vi "FrontPanelSingleChannel.vi"() -> ()   [LabVIEW 2017, in "LD Reading.lvclass"]
uses:
  LD Reading.lvclass
  Experimental Parameters.ctl
  Reference Channel Intensities.ctl
  Sample Channel Intensities.ctl
  Realtime Output.ctl
  Average Data.ctl
  AmplifierSettings.ctl
  LD Reading.lvclass/LD Reading.ctl
  MCTypedef.ctl
  <vilib>/Instr/_visa.llb/VISA Configure Serial Port (Instr).vi
  <vilib>/Utility/file.llb/Write Delimited Spreadsheet (string).vi
  <vilib>/Utility/inputDevices.llb/keyboardAcquire.vi
panel:
  in  "Experimental Controls":T1(tab)
  in  "Measure Dark Current":bool
  in  "Collect Data":bool
  out "Running":bool
  in  "Save Measurements?":bool
  in  "Stop and Discard \nMeasurement":bool
  in  "Output Filename (stem)":path
  out "Finished":bool
  in  "Data Collection Mode":enum32{"Reference", "Sample"}(radio)
  in  "Export Data":bool
  in  "Experimental Parameters":T2={"Correction Factor"=2.9405, "Data Interval (s)"=1.0, "Number of Data Points"=60.0, "Incident Angle (Degrees)"=63.0, "Refractive Index (Rare)"=1.335, "Refractive Index (Dense)"=1.55222, "PMT Bias Voltage (V)"=0.0, "Laser Wavelength (nm)"=0.0, "Preamplifier Output Gain (uA/V)"=10.0, "PEM Monitoring Frequency"=2} {"PEM Monitoring Frequency" min=1 max=2 step=1}
  in  "stop":bool
  out "read buffer":string
  in  "sp33d":dbl(knob)=0.5 step=0.5 scale=0.5..1.0
  in  "clear":bool
  out "error out":errorcluster
  out "Status":string
  out "Data Collection Progress":u8(slide) scale=0.0..100.0
  out "Reference Amplifier Settings":T3
  out "Signal Amplifier Settings":T3
  out "Corrected Signal":cluster{dbl[], dbl[]}(graph)
  out "RMS Voltage":cluster{dbl[], dbl[]}(graph)
  out "Signal PMT Voltage":cluster{dbl[], dbl[]}(graph)
  out "Reference PMT Voltage":cluster{dbl[], dbl[]}(graph)
  out "Realtime Output":T4
  out "Reference Averages":T5
  out "Sample Averages":T5
  out "Reference Analysis":T6
  out "Sample Analysis":T7
  # "Dichroism Controller"
  # "Translation Stage Controls"
  # "Data Collection Parameters"
  # "System Settings"
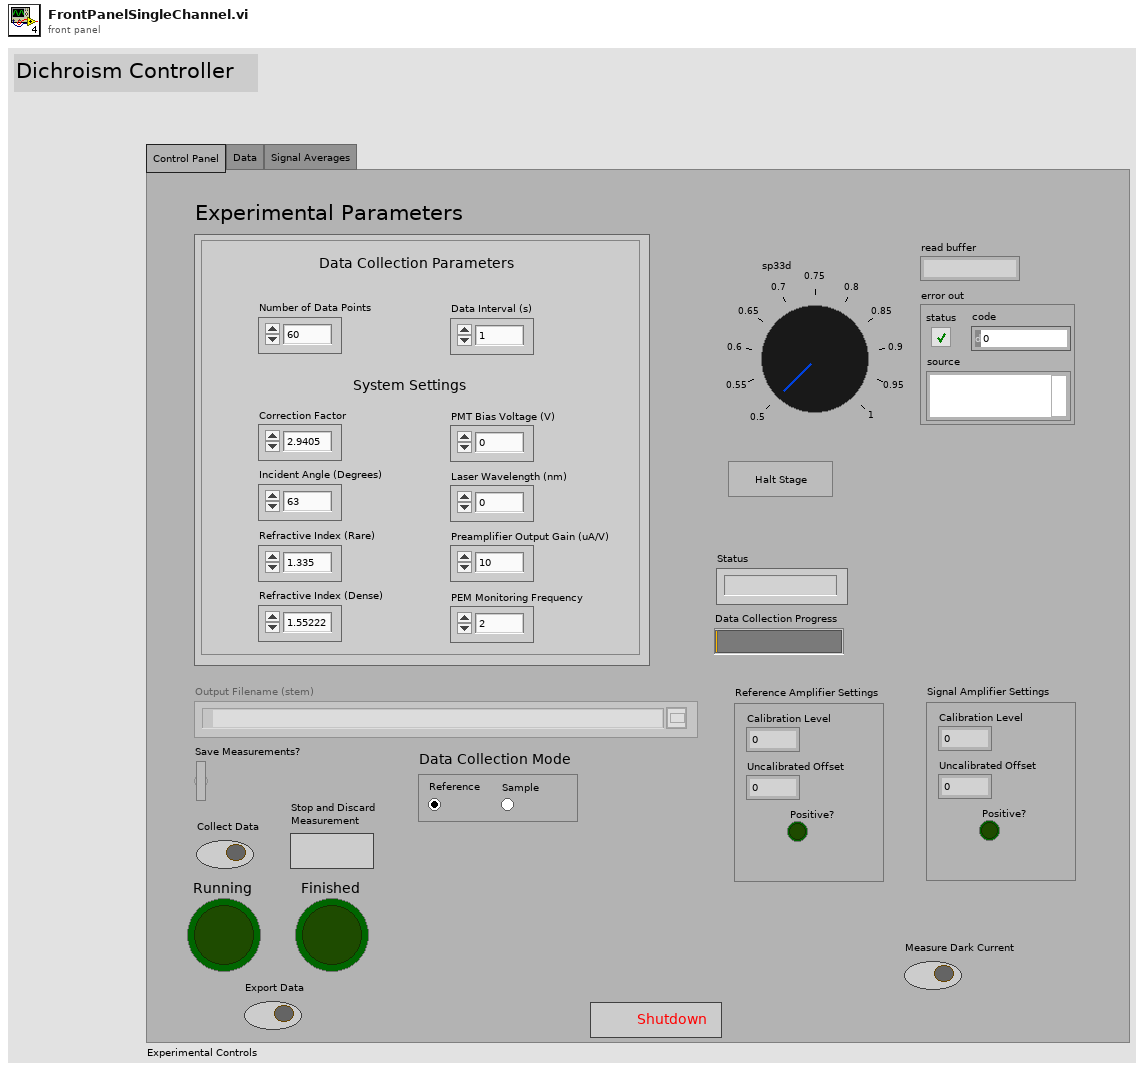
[diagram p1: front panel]
types:
  T1 = enum32{"Control Panel", "Data", "Signal Averages"}
  T2 = typedef "Experimental Parameters.ctl" = cluster{"Correction Factor":dbl, "Data Interval (s)":dbl, "Number of Data Points":dbl, "Incident Angle (Degrees)":dbl, "Refractive Index (Rare)":dbl, "Refractive Index (Dense)":dbl, "PMT Bias Voltage (V)":dbl, "Laser Wavelength (nm)":dbl, "Preamplifier Output Gain (uA/V)":dbl, "PEM Monitoring Frequency":u8}
  T3 = typedef "AmplifierSettings.ctl" = cluster{"Calibration Level":dbl, "Uncalibrated Offset":dbl, "Positive?":bool}
  T4 = typedef "Realtime Output.ctl" = cluster{"Elapsed Time (s)":dbl, "PMT Voltage (V)":dbl, "Diode Voltage (V)":dbl, "RMS Voltage (V)":dbl, "Theta (Degrees)":dbl, "PEM Frequency (Hz)":dbl}
  T5 = typedef "Average Data.ctl" = cluster{"Data":cluster{"Signal PMT Voltage (V)":dbl, "Reference PMT Voltage (V)":dbl, "RMS Voltage (V)":dbl, "Theta (Degrees)":dbl}}
  T6 = typedef "Reference Channel Intensities.ctl" = cluster{"Data":cluster{"I_par":dbl, "I_perp":dbl}}
  T7 = typedef "Sample Channel Intensities.ctl" = cluster{"Data":cluster{"I_par":dbl, "I_perp":dbl, "Dichroic Ratio":dbl, "Angle (Degrees)":dbl}}
  T8 = enum8{"Enabled", "Disabled", "Disabled and Grayed Out"}
  T9 = typedef "MCTypedef.ctl" = enum16{"idle", "forward", "reverse", "clear"}
  T10 = cluster{dbl[], dbl[], dbl[], dbl[], dbl[], dbl[], dbl[]}
  T11 = cluster{"RMS Voltage Array":dbl[], "Photodiode Voltage Array":dbl[], "PMT Voltage Array":dbl[], "Diode/PMT Ratio Array":dbl[], "Time Array":dbl[], "PEM Frequency Array":dbl[], "Theta Array":dbl[]}
  T12 = cluster{"Signal PMT Voltage (V)":dbl, "Reference PMT Voltage (V)":dbl, "RMS Voltage (V)":dbl, "Theta (Degrees)":dbl}
  T13 = cluster{"I_par":dbl, "I_perp":dbl, "Dichroic Ratio":dbl, "Angle (Degrees)":dbl}
  T14 = typedef "NI_Matrix.lvlib/RealMatrix.ctl" = dbl[][]
  T15 = enum16{"0", "1", "2", "3", "4", "5", "6", "7", "8", "9", "A", "B", "C", "D", "E", "F", "G", "H", "I", "J", "K", "L", "M", "N", "O", "P", "Q", "R", "S", "T", "U", "V", "W", "X", "Y", "Z", "F1", "F2", "F3", "F4", "F5", "F6", "F7", "F8", "F9", "F10", "F11", "F12", "F13", "F14", "F15", "ADD", "BACK", "BACKSLASH", "CAPITAL", "COMMA", "DECIMAL", "DELETE", "DIVIDE", "DOWN", "END", "EQUALS", "ESCAPE", "GRAVE (`)", "HOME", "INSERT", "LBRACKET", "LCONTROL", "LEFT", "L ALT", "LSHIFT", "LWIN", "MINUS", "MULTIPLY", "NEXT", "NUMLOCK", "NUMPAD_0", "NUMPAD_1", "NUMPAD_2", "NUMPAD_3", "NUMPAD_4", "NUMPAD_5", "NUMPAD_6", "NUMPAD_7", "NUMPAD_8", "NUMPAD_9", "PAUSE", "PERIOD", "PRIOR (PG UP)", "RBRACKET", "RCONTROL", "RETURN", "RIGHT", "R ALT", "RSHIFT", "RWIN", "SCROLL", "SEMICOLON", "SLASH", "SPACE", "SUBTRACT", "TAB", "UP", "ENTER (num pad)", "' (quote)"}[]
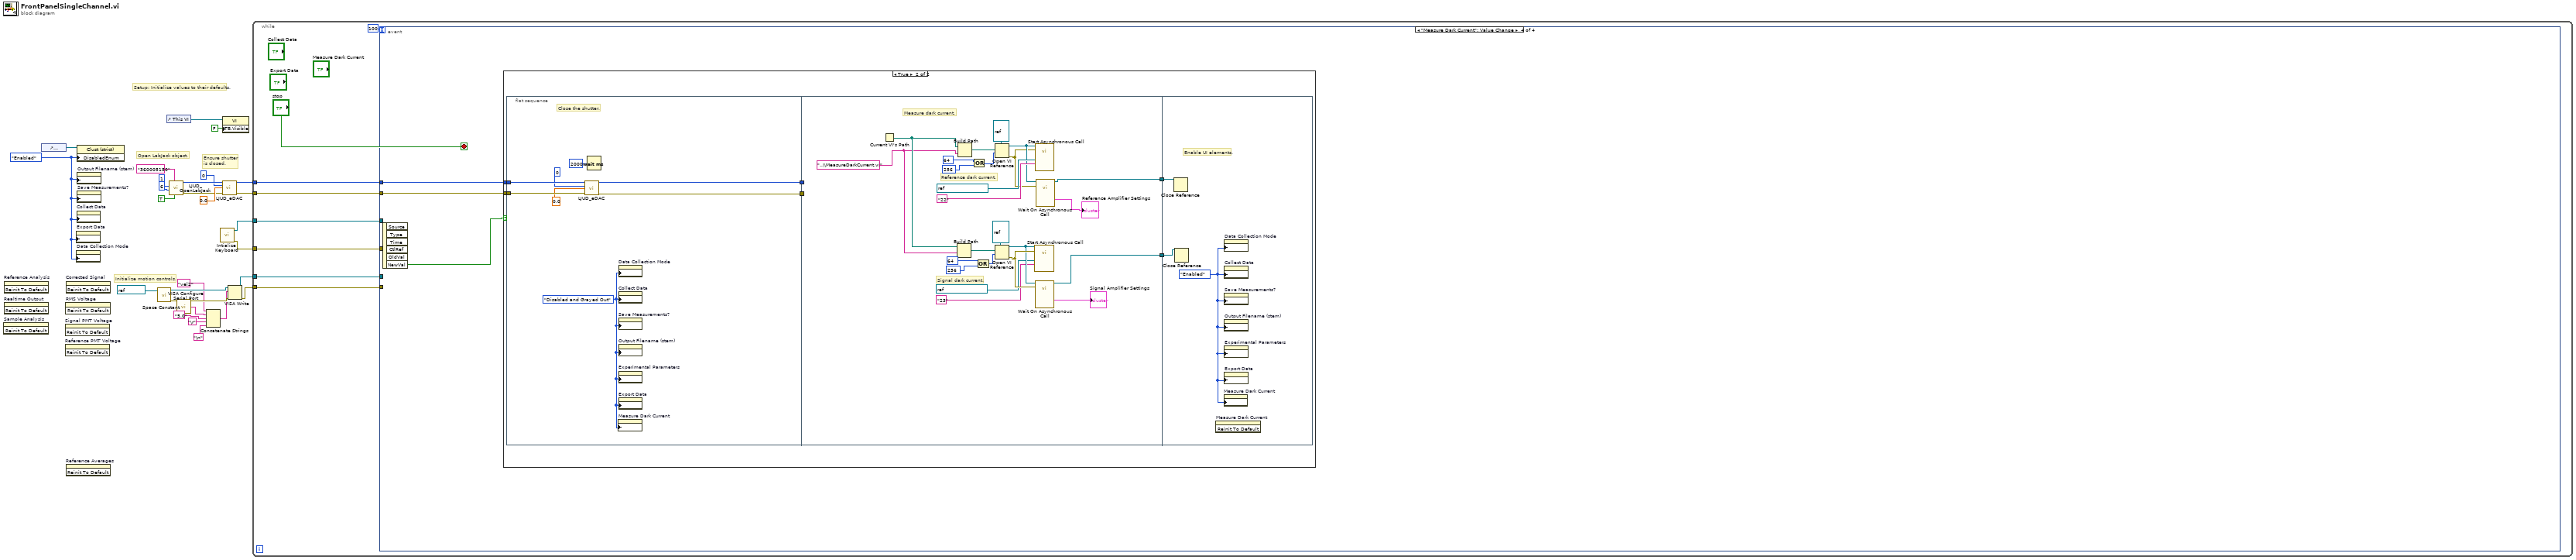
[diagram p0: block diagram]
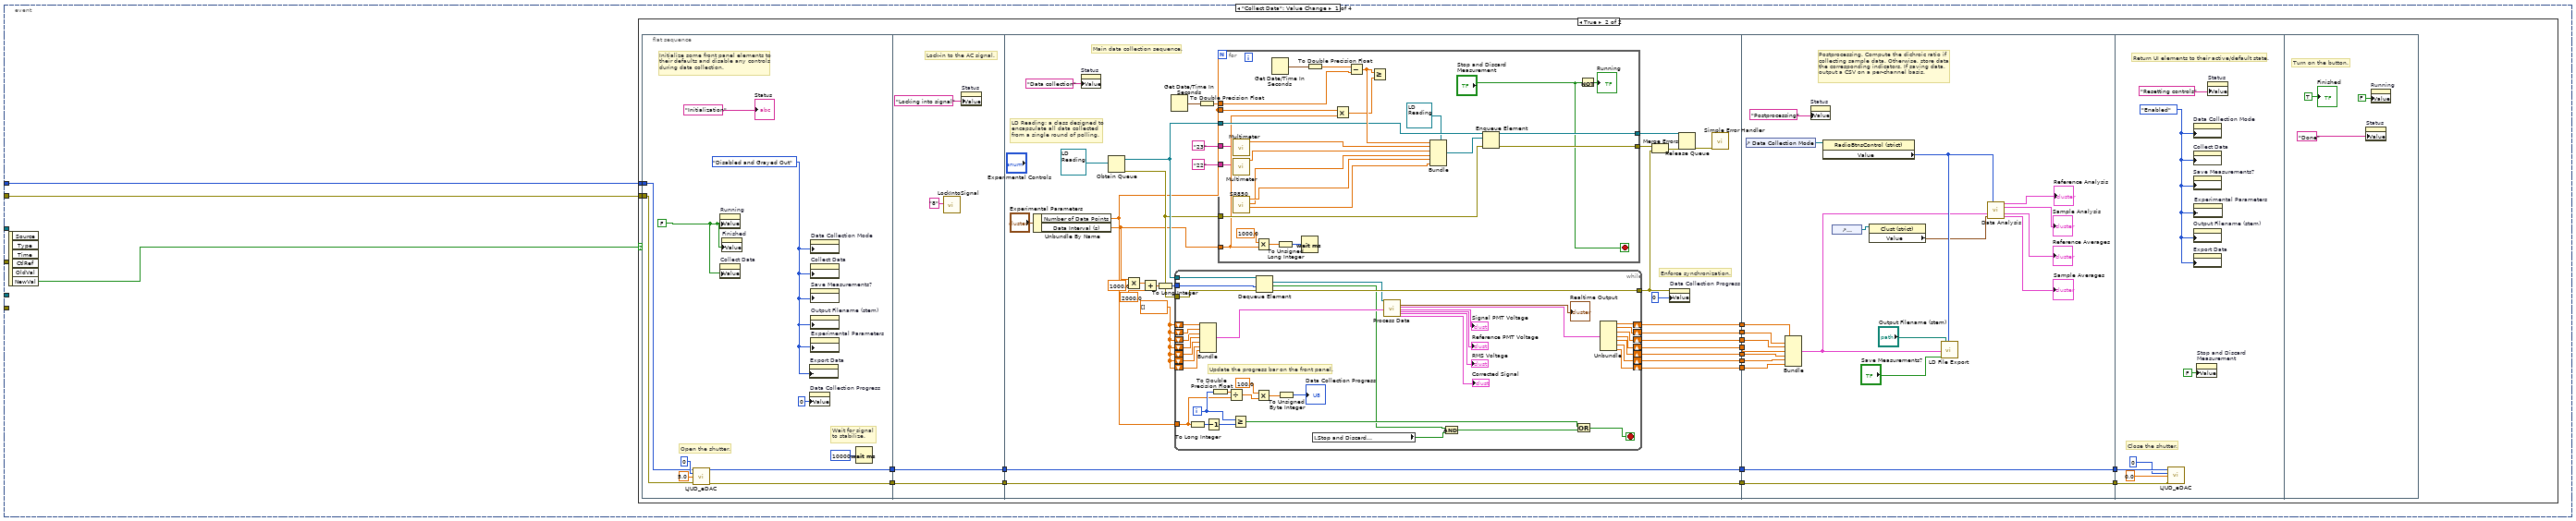
[diagram p2: hidden frame]
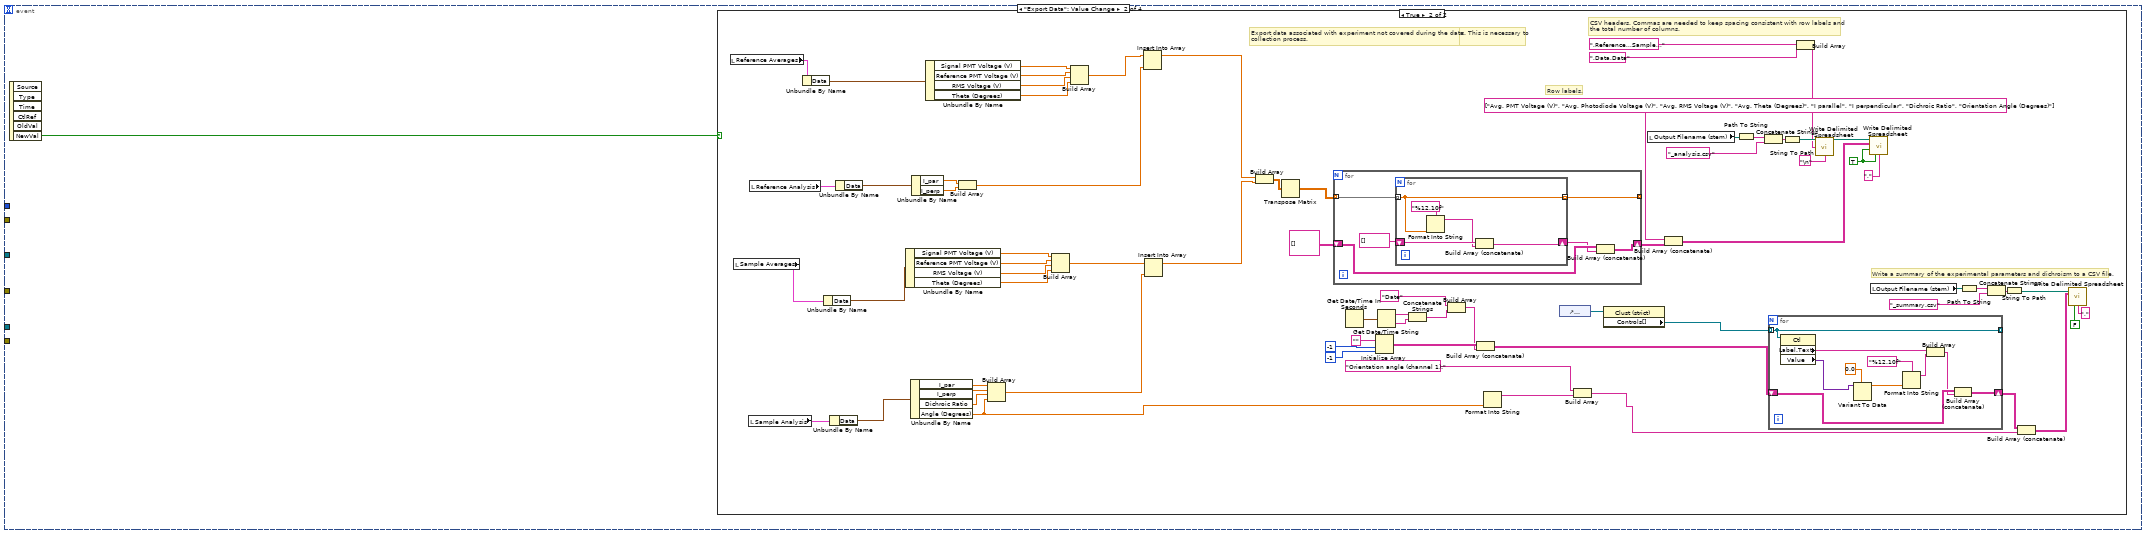
[diagram p4: hidden frame]
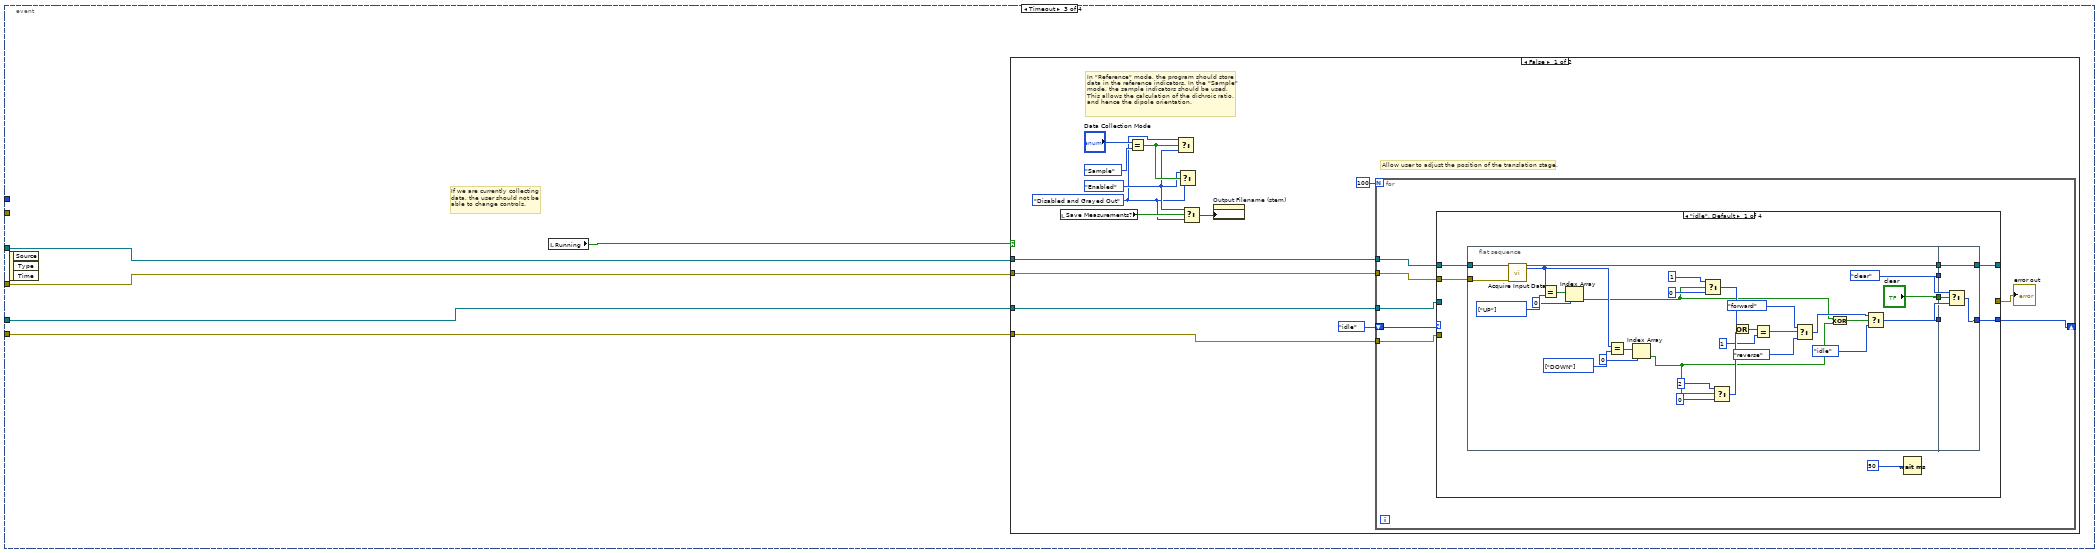
[diagram p6: hidden frame]
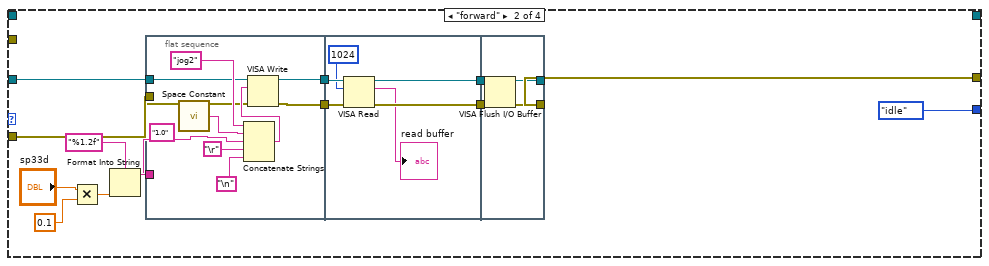
[diagram p7: hidden frame]
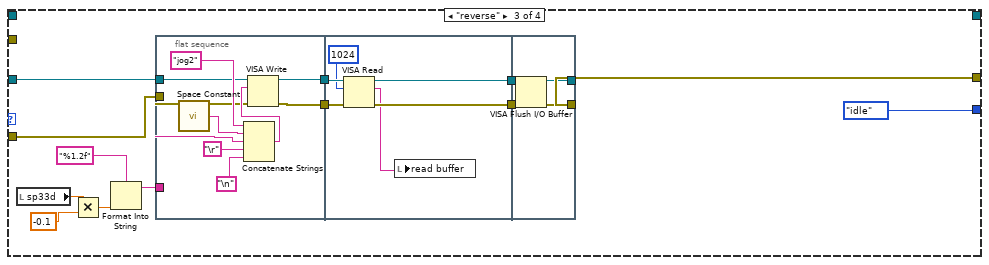
[diagram p8: hidden frame]
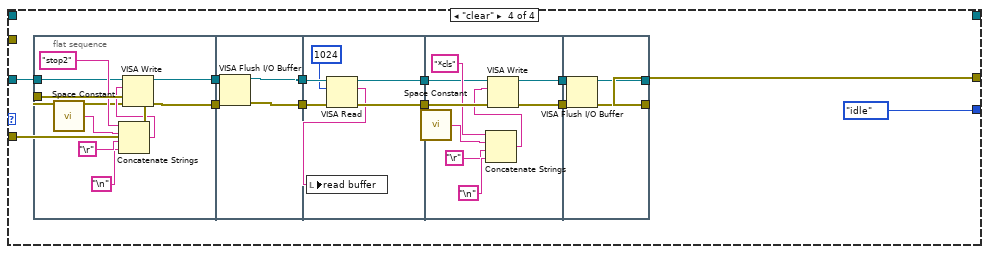
[diagram p9: hidden frame]
diagram:
  w24 = T8."Enabled" ("Disabled")
  # "Ensure shutter\nis closed."
  # "Open LabJack object."
  # "Initialize motion controls."
  # "Setup: Initialize values to their defaults."
  n1 = invoke on="Sample Analysis" class="Clust (strict)" method="Reinit To Default"() -> ()  [unwired: 3 in, 3 out]
  n2 = invoke on="Reference Analysis" class="Clust (strict)" method="Reinit To Default"() -> ()  [unwired: 3 in, 3 out]
  n3 = invoke on="Realtime Output" class="Clust (strict)" method="Reinit To Default"() -> ()  [unwired: 3 in, 3 out]
  n4 = control-ref of="Experimental Parameters"() -> (w25:refnum<vi>)
  n5 = invoke on="Signal PMT Voltage" class="XYGraph (strict)" method="Reinit To Default"() -> ()  [unwired: 3 in, 3 out]
  n6 = invoke on="Reference PMT Voltage" class="XYGraph (strict)" method="Reinit To Default"() -> ()  [unwired: 3 in, 3 out]
  n7 = invoke on="RMS Voltage" class="XYGraph (strict)" method="Reinit To Default"() -> ()  [unwired: 3 in, 3 out]
  n8 = invoke on="Corrected Signal" class="XYGraph (strict)" method="Reinit To Default"() -> ()  [unwired: 3 in, 3 out]
  n9 = invoke on="Reference Averages" class="Clust (strict)" method="Reinit To Default"() -> ()  [unwired: 3 in, 3 out]
  n10 = property on="Export Data" class="Bool"("DisabledEnum"=w24) -> ()  [unwired: 2 in, 2 out]
  n11 = property on="Data Collection Mode" class="RadioBtnsControl (strict)"("DisabledEnum"=w24) -> ()  [unwired: 2 in, 2 out]
  n12 = property class="Clust (strict)"(reference=w25, "DisabledEnum"=w24) -> ()  [unwired: 1 in, 2 out]
  n13 = property on="Collect Data" class="Bool (strict)"("DisabledEnum"=w24) -> ()  [unwired: 2 in, 2 out]
  n14 = property on="Output Filename (stem)" class="Path"("DisabledEnum"=w24) -> ()  [unwired: 2 in, 2 out]
  n15 = property on="Save Measurements?" class="Bool (strict)"("DisabledEnum"=w24) -> ()  [unwired: 2 in, 2 out]
  n16 = call-poly "VISA Configure Serial Port"("VISA resource name"=refnum<visa-resource-name> "COM1") -> ("VISA resource name out"=w22:refnum<visa-resource-name>, "error out"=w23:errorcluster)  [unwired: 13 in]
  n17 = control-ref of="This VI"() -> (w26:refnum<vi>)
  n18 = call "LJUD_OpenLabJack.vi"("FirstFound"=TRUE, "Address"="360005150", "ConnectionType"=1, "DeviceType"=6) -> ("error out"=w1:errorcluster, "Handle"=w6:i32)  [unwired: 6 in]
  n19 = call <vilib>:"Space Constant.vi"() -> ("String"=w21:string)
  n20 = Concatenate Strings("vel2" ("string"), w21, "5.0" ("string"), "\r", "\n") -> (w20:string)
  n21 = call <vilib>:"Intialize Keyboard.vi"() -> ("error out"=w12:errorcluster, "device ID"=w11:refnum<k1>)  [unwired: 10 in]
  n22 = property class="VI"(reference=w26, "TB.Visible"=FALSE ("Tool Bar:Visible")) -> ()  [unwired: 1 in, 2 out]
  n23 = call "LJUD_eDAC.vi"("Handle In"=w6, "Channel"=0, "Voltage"=0.0, "error in"=w1) -> ("Handle Out"=w5:i32, "error out"=w4:errorcluster)  [unwired: 10 in]
  n24 = VISA Write(VISA resource name=w22, write buffer=w20, error in (no error)=w23) -> (VISA resource name out=w13:refnum<visa-resource-name>, error out=w14:errorcluster)  [unwired: 1 out]
  n25 = while {
    tunnel: w14 -> [w33]
    tunnel: w13 -> [w32]
    tunnel: w12 -> [w31]
    tunnel: w11 -> [w30]
    tunnel: w5 -> [w29]
    tunnel: w4 -> [w28]
    stop <- "stop" stop-if-true
    n26 = event shown="[3] \"Measure Dark Current\": Value Change" {
      selector: _ -> [_ _ _ _]
      dyn-events: _ -> [_ _ _ _]
      timeout: 100 -> [_ _ _ _]
      tunnel: w33 -> [_ _ w295 _]
      tunnel: w32 -> [_ _ w294 _]
      tunnel: w31 -> [_ _ w293 _]
      tunnel: w30 -> [_ _ w292 _]
      tunnel: w29 -> [w37 _ _ w471]
      tunnel: w28 -> [w36 _ _ w470]
      event "Collect Data": Value Change {
        n27 = event-data() -> ("NewVal"=w38:bool)  [unwired: 1 in, 5 out]
        n28 = case shown="True" w38 {
          tunnel: w37 -> [_ w48]
          tunnel: w36 -> [_ w47]
          frame False {
          }
          frame True {
            n29 = flat-sequence {
              tunnel: w48 -> [w60]
              tunnel: w47 -> [w59]
              tunnel: [w58] -> w42
              tunnel: [w57] -> w40
              tunnel: w42 -> [w70]
              tunnel: [w70] -> w41
              tunnel: w40 -> [w69]
              tunnel: [w69] -> w39
              tunnel: [w92] -> w55
              tunnel: [w91] -> w54
              tunnel: [w90] -> w53
              tunnel: [w93] -> w52
              tunnel: [w89] -> w51
              tunnel: [w88] -> w50
              tunnel: [w83] -> w49
              tunnel: [w72] -> w45
              tunnel: w41 -> [w72]
              tunnel: [w71] -> w43
              tunnel: w39 -> [w71]
              tunnel: w55 -> [w184]
              tunnel: w54 -> [w183]
              tunnel: w53 -> [w182]
              tunnel: w52 -> [w185]
              tunnel: w51 -> [w181]
              tunnel: w50 -> [w180]
              tunnel: w49 -> [w179]
              tunnel: [w169] -> w46
              tunnel: w45 -> [w169]
              tunnel: [w168] -> w44
              tunnel: w43 -> [w168]
              tunnel: w46 -> [w192]
              tunnel: w44 -> [w191]
              frame #0 {
                w63 = T8."Disabled and Grayed Out" ("Disabled")
                w64 = FALSE
                # "Wait for signal \nto stabilize."
                # "Open the shutter."
                # "Initialize some front panel elements to \ntheir defaults and disable any controls \nduring data collection."
                n30 = call "LJUD_eDAC.vi"("Handle In"=w60, "Channel"=0, "Voltage"=5.0, "error in"=w59) -> ("Handle Out"=w58:i32, "error out"=w57:errorcluster)  [unwired: 10 in]
                n31 = property on="Running" class="Bool (strict)"("Value"=w64) -> ()  [unwired: 2 in, 2 out]
                n32 = property on="Collect Data" class="Bool (strict)"("Value"=w64) -> ()  [unwired: 2 in, 2 out]
                n33 = property on="Finished" class="Bool (strict)"("Value"=w64) -> ()  [unwired: 2 in, 2 out]
                n34 = property on="Export Data" class="Bool"("DisabledEnum"=w63) -> ()  [unwired: 2 in, 2 out]
                n35 = property on="Data Collection Progress" class="Slide (strict)"("Value"=u8 0 ("Progress")) -> ()  [unwired: 2 in, 2 out]
                n36 = property on="Data Collection Mode" class="RadioBtnsControl (strict)"("DisabledEnum"=w63) -> ()  [unwired: 2 in, 2 out]
                n37 = property on="Collect Data" class="Bool (strict)"("DisabledEnum"=w63) -> ()  [unwired: 2 in, 2 out]
                n38 = property on="Save Measurements?" class="Bool (strict)"("DisabledEnum"=w63) -> ()  [unwired: 2 in, 2 out]
                n39 = property on="Output Filename (stem)" class="Path"("DisabledEnum"=w63) -> ()  [unwired: 2 in, 2 out]
                n40 = property on="Experimental Parameters" class="Clust (strict)"("DisabledEnum"=w63) -> ()  [unwired: 2 in, 2 out]
                n41 = Wait (ms)(milliseconds to wait=u32 10000) -> ()  [unwired: 1 out]
                "Status" <- "Initialization"
              }
              frame #1 {
                # "Lock-in to the AC signal."
                n42 = call "LockIntoSignal.vi"("GPIB Address"="8") -> ()  [unwired: 10 in, 1 out]
                n43 = property on="Status" class="Str"("Value"="Locking into signal") -> ()  [unwired: 2 in, 2 out]
              }
              frame #2 {
                w84 = dbl[] []
                # "Enforce synchronization."
                # "Main data collection sequence."
                # "LD Reading: a class designed to \nencapsulate all data collected \nfrom a single round of polling."
                n44 = Unbundle By Name("Experimental Parameters") -> ("Number of Data Points"=w81:dbl, "Data Interval (s)"=w80:dbl)
                n45 = property on="Status" class="Str"("Value"="Data collection") -> ()  [unwired: 2 in, 2 out]
                n46 = Obtain Queue(element data type=refnum<class "LD Reading.lvclass"> refnum ("LD Reading.lvclass")) -> (queue out=w99:refnum<queue>, error out=w98:errorcluster)  [unwired: 4 in, 1 out]
                n47 = Multiply(x=w80, y=1000.0) -> (x*y=w78:dbl)
                n48 = Add(x=w78, y=2000.0) -> (x+y=w76:dbl)
                n49 = To Long Integer(number=w76) -> (32bit integer=w75:i32)
                n50 = Get Date/Time In Seconds() -> (seconds since 1Jan1904=w102:timestamp)
                n51 = while {
                  tunnel: w99 -> [w167]
                  shift-right: [w146] -> w93
                  shift-left: w84 -> [w153]
                  shift-right: [w145] -> w92
                  shift-left: w84 -> [w152]
                  shift-right: [w144] -> w91
                  shift-left: w84 -> [w151]
                  shift-right: [w143] -> w90
                  shift-left: w84 -> [w150]
                  shift-right: [w142] -> w89
                  shift-left: w84 -> [w149]
                  shift-right: [w141] -> w88
                  shift-left: w84 -> [w148]
                  shift-right: [w140] -> w83
                  shift-left: w84 -> [w147]
                  tunnel: w98 -> [w165]
                  tunnel: [w164] -> w86
                  tunnel: w81 -> [w154]
                  tunnel: w75 -> [w128]
                  i -> [w159]
                  stop <- w166 stop-if-true
                  # "Update the progress bar on the front panel."
                  n52 = To Long Integer(number=w154) -> (32bit integer=w160:i32)
                  n53 = Bundle(w153, w152, w151, w150, w149, w148, w147) -> (w138:T10)  [unwired: 1 in]
                  n54 = Decrement(x=w160) -> (x-1=w163:i32)
                  n55 = To Double Precision Float(number=w159) -> (double precision float=w158:dbl)
                  n56 = Divide(x=w158, y=w154) -> (x/y=w161:dbl)
                  n57 = Greater Or Equal?(x=w159, y=w163) -> (x >= y?=w162:bool)
                  n58 = Multiply(x=100.0, y=w161) -> (x*y=w156:dbl)
                  n59 = Dequeue Element(queue=w167, timeout in ms (-1)=w128, error in (no error)=w165) -> (element=w139:refnum<class "LD Reading.lvclass">, timed out?=w131:bool, error out=w164:errorcluster)  [unwired: 1 out]
                  n60 = To Unsigned Byte Integer(number=w156) -> (unsigned 8bit integer=→"Data Collection Progress":u8)
                  n61 = local read "Stop and Discard \nMeasurement"() -> (w130:bool)
                  n62 = call "Process Data.vi"("LD Reading in"=w139, "Input Cluster"=w138) -> ("Realtime Output"=→"Realtime Output":T4, "Output Cluster"=w136:T11, "PMT Voltage (V)"=→"Signal PMT Voltage":cluster{dbl[], dbl[]}, "Photodiode Voltage  (V)"=→"Reference PMT Voltage":cluster{dbl[], dbl[]}, "RMS Voltage (mV)"=→"RMS Voltage":cluster{dbl[], dbl[]}, "Diode/PMT"=→"Corrected Signal":cluster{dbl[], dbl[]})  [unwired: 20 in]
                  n63 = And(x=w131, y=w130) -> (x .and. y?=w129:bool)
                  n64 = Or(x=w162, y=w129) -> (x .or. y?=w166:bool)
                  n65 = Unbundle(w136) -> ("RMS Voltage Array"=w146:dbl[], "Photodiode Voltage Array"=w145:dbl[], "PMT Voltage Array"=w144:dbl[], "Diode/PMT Ratio Array"=w143:dbl[], "Time Array"=w142:dbl[], "PEM Frequency Array"=w141:dbl[], "Theta Array"=w140:dbl[])
                }
                n66 = To Double Precision Float(number=w102) -> (double precision float=w101:dbl)
                n67 = for {
                  N: w81 -> [_]
                  tunnel: w80 -> [w108]
                  tunnel: w101 -> [w117]
                  tunnel: w99 -> [w124]
                  tunnel: [w121] -> w94
                  tunnel: w98 -> [w119]
                  tunnel: [w118] -> w97
                  tunnel: w81 -> [w116]
                  tunnel: "23" ("GPIB Address") -> [w105]
                  tunnel: "22" ("GPIB Address") -> [w103]
                  stop <- "Stop and Discard \nMeasurement" stop-if-true
                  n68 = call "Multimeter.vi"("GPIB Address"=w105) -> ("Voltage"=w111:dbl)  [unwired: 9 in, 1 out]
                  n69 = call "Multimeter.vi"("GPIB Address"=w103) -> ("Voltage"=w104:dbl)  [unwired: 9 in, 1 out]
                  n70 = call "SR850.vi"() -> ("Frequency"=w112:dbl, "R"=w113:dbl, "Theta"=w114:dbl)  [unwired: 8 in, 1 out]
                  n71 = Multiply(x=1000.0, y=w108) -> (x*y=w110:dbl)
                  n72 = Get Date/Time In Seconds() -> (seconds since 1Jan1904=w127:timestamp)
                  n73 = To Unsigned Long Integer(number=w110) -> (unsigned 32bit integer=w107:u32)
                  n74 = Wait (ms)(milliseconds to wait=w107) -> ()  [unwired: 1 out]
                  n75 = To Double Precision Float(number=w127) -> (double precision float=w126:dbl)
                  n76 = Multiply(x=w116, y=w108) -> (x*y=w115:dbl)
                  n77 = Subtract(x=w126, y=w117) -> (x-y=w125:dbl)
                  n78 = Greater Or Equal?(x=w125, y=w115) -> ()  [unwired: 1 out]
                  n79 = Bundle(cluster=refnum<class "LD Reading.lvclass"> refnum ("LD Reading.lvclass"), w125, w111, w104, w113, w114, w112) -> (w122:refnum<class "LD Reading.lvclass">)
                  n80 = Enqueue Element(queue=w124, element=w122, error in (no error)=w119) -> (queue out=w121:refnum<queue>, error out=w118:errorcluster)  [unwired: 1 in, 1 out]
                  n81 = Not(x="Stop and Discard \nMeasurement") -> (.not. x?=→"Running":bool)
                }
                n82 = Merge Errors(w97, w86) -> (w96:errorcluster)
                n83 = property on="Data Collection Progress" class="Slide (strict)"(error in=w86, "Value"=u8 0 ("Progress")) -> ()  [unwired: 1 in, 2 out]
                n84 = Release Queue(queue=w94, error in (no error)=w96) -> (error out=w95:errorcluster)  [unwired: 1 in, 2 out]
                n85 = call <vilib>:"Simple Error Handler.vi"("error in (no error)"=w95) -> ()  [unwired: 4 in, 5 out]
              }
              frame #3 {
                # "Postprocessing. Compute the dichroic ratio if \ncollecting sample data. Otherwise, store data \nthe corresponding indicators. If saving data, \noutput a CSV on a per-channel basis."
                n86 = control-ref of="Data Collection Mode"() -> (w178:refnum<vi>)
                n87 = Bundle(w185, w184, w183, w182, w181, w180, w179) -> (w172:T10)  [unwired: 1 in]
                n88 = property on="Status" class="Str"("Value"="Postprocessing") -> ()  [unwired: 2 in, 2 out]
                n89 = property class="RadioBtnsControl (strict)"(reference=w178) -> ("Value"=w173:enum32{"Reference", "Sample"})  [unwired: 1 in, 2 out]
                n90 = control-ref of="Experimental Parameters"() -> (w171:refnum<vi>)
                n91 = property class="Clust (strict)"(reference=w171) -> ("Value"=w170:T2)  [unwired: 1 in, 2 out]
                n92 = call "LD File Export.vi"("Input Cluster"=w172, "Save Data?"="Save Measurements?", "Output Filename (stem)"="Output Filename (stem)", "Data Collection Mode"=w173) -> ()  [unwired: 16 in]
                n93 = call "Data Analysis.vi"("Data Collection Mode"=w173, "Cluster"=w172, "Experimental Parameters"=w170) -> ("Reference Analysis"=→"Reference Analysis":T6, "Sample Analysis"=→"Sample Analysis":T7, "Reference Averages"=→"Reference Averages":T5, "Sample Averages"=→"Sample Averages":T5)  [unwired: 9 in]
              }
              frame #4 {
                w193 = T8."Enabled" ("Disabled")
                # "Close the shutter."
                # "Return UI elements to their active/default state."
                n94 = call "LJUD_eDAC.vi"("Handle In"=w192, "Channel"=0, "Voltage"=0.0, "error in"=w191) -> ()  [unwired: 10 in, 2 out]
                n95 = property on="Data Collection Mode" class="RadioBtnsControl (strict)"("DisabledEnum"=w193) -> ()  [unwired: 2 in, 2 out]
                n96 = property on="Collect Data" class="Bool (strict)"("DisabledEnum"=w193) -> ()  [unwired: 2 in, 2 out]
                n97 = property on="Save Measurements?" class="Bool (strict)"("DisabledEnum"=w193) -> ()  [unwired: 2 in, 2 out]
                n98 = property on="Output Filename (stem)" class="Path"("DisabledEnum"=w193) -> ()  [unwired: 2 in, 2 out]
                n99 = property on="Export Data" class="Bool"("DisabledEnum"=w193) -> ()  [unwired: 2 in, 2 out]
                n100 = property on="Experimental Parameters" class="Clust (strict)"("DisabledEnum"=w193) -> ()  [unwired: 2 in, 2 out]
                n101 = property on="Stop and Discard \nMeasurement" class="Bool (strict)"("Value"=FALSE ("Stop Data Collection")) -> ()  [unwired: 2 in, 2 out]
                n102 = property on="Status" class="Str"("Value"="Resetting controls") -> ()  [unwired: 2 in, 2 out]
              }
              frame #5 {
                # "Turn on the button."
                n103 = property on="Status" class="Str"("Value"="Done") -> ()  [unwired: 2 in, 2 out]
                n104 = property on="Running" class="Bool (strict)"("Value"=FALSE ("Running")) -> ()  [unwired: 2 in, 2 out]
                "Finished" <- TRUE ("Finished")
              }
            }
          }
        }
      }
      event "Export Data": Value Change {
        n105 = event-data() -> ("NewVal"=w199:bool)  [unwired: 1 in, 5 out]
        n106 = case shown="True" w199 {
          frame False {
          }
          frame True {
            w231 = TRUE ("append to file? (new file:F)")
            # "Write a summary of the experimental parameters and dichroism to a CSV file."
            # "CSV headers. Commas are needed to keep spacing consistent with row labels and \nthe total number of columns."
            # "Convert matrix of doubles into a matrix of properly formatted strings. This is necessary to \nprepend the row labels, which are strings."
            # "Row labels."
            # "Export data associated with experiment not covered during the data \ncollection process."
            n107 = local read "Reference Averages"() -> (w265:T5)
            n108 = local read "Sample Averages"() -> (w264:T5)
            n109 = local read "Sample Analysis"() -> (w262:T7)
            n110 = local read "Reference Analysis"() -> (w267:T6)
            n111 = Unbundle By Name(w265) -> ("Data"=w202:T12)
            n112 = Unbundle By Name(w264) -> ("Data"=w249:T12)
            n113 = Unbundle By Name(w262) -> ("Data"=w263:T13)
            n114 = Unbundle By Name(w267) -> ("Data"=w266:cluster{"I_par":dbl, "I_perp":dbl})
            n115 = Unbundle By Name(w249) -> ("Signal PMT Voltage (V)"=w250:dbl, "Reference PMT Voltage (V)"=w251:dbl, "RMS Voltage (V)"=w252:dbl, "Theta (Degrees)"=w253:dbl)
            n116 = Unbundle By Name(w263) -> ("I_par"=w248:dbl, "I_perp"=w247:dbl, "Dichroic Ratio"=w224:dbl, "Angle (Degrees)"=w203:dbl)
            n117 = Unbundle By Name(w266) -> ("I_par"=w255:dbl, "I_perp"=w254:dbl)
            n118 = Unbundle By Name(w202) -> ("Signal PMT Voltage (V)"=w259:dbl, "Reference PMT Voltage (V)"=w258:dbl, "RMS Voltage (V)"=w257:dbl, "Theta (Degrees)"=w256:dbl)
            n119 = Build Array(w255, w254) -> (w246:dbl[])
            n120 = Build Array(w248, w247, w224, w203) -> (w244:dbl[])
            n121 = Build Array(w250, w251, w252, w253) -> (w245:dbl[])
            n122 = Build Array(w259, w258, w257, w256) -> (w201:dbl[])
            n123 = Insert Into Array(array=w201, new element=w246) -> (w243:dbl[])  [unwired: 1 in]
            n124 = Insert Into Array(array=w245, new element=w244) -> (w200:dbl[])  [unwired: 1 in]
            n125 = Build Array(w243, w200) -> (w236:T14)
            n126 = Transpose Matrix(1:w236) -> (0:w230:T14)
            n127 = for {
              tunnel: w230 -> [w286] mode=indexing
              tunnel: [w285] -> _ mode=indexing
              shift-right: [w281] -> w233
              shift-left: string[][] [] -> [w283]
              n128 = for {
                tunnel: w286 -> [w291] mode=indexing
                tunnel: [w291] -> w285 mode=indexing
                shift-right: [w287] -> w282
                shift-left: string[] [] -> [w289]
                n129 = Format Into String(format string="%12.10f", w291) -> (resulting string=w288:string)  [unwired: 2 in, 1 out]
                n130 = Build Array (concatenate)(w289, w288) -> (w287:string[])
              }
              n131 = Build Array (concatenate)(w283, w282) -> (w281:string[][])
            }
            n132 = Get Date/Time In Seconds() -> (seconds since 1Jan1904=w221:timestamp)
            n133 = Initialize Array("", -1 ("dimension size"), -1 ("dimension size")) -> (w214:string[][])
            n134 = Get Date/Time String(seconds (now)=w221) -> (date string=w220:string, time string=w219:string)  [unwired: 2 in]
            n135 = Concatenate Strings(w220, w219) -> (w217:string)
            n136 = Build Array("Date", w217) -> (w213:string[])
            n137 = Build Array (concatenate)(w214, w213) -> (w209:string[][])
            n138 = Format Into String(w203) -> (resulting string=w212:string)  [unwired: 3 in, 1 out]
            n139 = control-ref of="Experimental Parameters"() -> (w223:refnum<vi>)
            n140 = Build Array("Orientation angle (channel 1):", w212) -> (w210:string[])
            n141 = property class="Clust (strict)"(reference=w223) -> ("Controls[]"=w222:refnum<vi>[])  [unwired: 1 in, 2 out]
            n142 = local read "Output Filename (stem)"() -> (w270:path)
            n143 = Build Array (concatenate)(string[] ["Avg. PMT Voltage (V)", "Avg. Photodiode Voltage (V)", "Avg. RMS Voltage (V)", "Avg. Theta (Degrees)", "I parallel", "I perpendicular", "Dichroic Ratio", "Orientation Angle (Degrees)"], w233) -> (w232:string[][])
            n144 = Path To String(path=w270) -> (string=w269:string)
            n145 = Concatenate Strings(w269, "_analysis.csv") -> (w261:string)
            n146 = for {
              tunnel: w222 -> [w280] mode=indexing
              tunnel: [w280] -> _ mode=indexing
              shift-right: [w274] -> w208
              shift-left: w209 -> [w278]
              n147 = property class="Ctl"(reference=w280) -> ("Label.Text"=w277:string, "Value"=w273:variant)  [unwired: 1 in, 2 out]
              n148 = Variant To Data(type=0.0, Variant=w273) -> (data=w271:dbl)  [unwired: 1 in, 1 out]
              n149 = Format Into String(format string="%12.10f", w271) -> (resulting string=w276:string)  [unwired: 2 in, 1 out]
              n150 = Build Array(w277, w276) -> (w275:string[])
              n151 = Build Array (concatenate)(w278, w275) -> (w274:string[][])
            }
            n152 = String To Path(string=w261) -> (path=w260:path)
            n153 = Build Array(",Reference,,,Sample,,,", ",Data,Data") -> (w238:string[])
            n154 = call-poly <vilib>:"Write Delimited Spreadsheet.vi"("file path (dialog if empty)"=w260, "1D data"=w238, "delimiter (\\t)"="\n" ("delimiter (\\t)")) -> ("new file path (Not A Path if cancelled)"=w242:path)  [unwired: 11 in, 1 out]
            n155 = call-poly <vilib>:"Write Delimited Spreadsheet.vi"("file path (dialog if empty)"=w242, "2D data"=w232, "append to file? (new file:F)"=w231, "transpose? (no:F)"=w231, "delimiter (\\t)"="," ("delimiter (\\t)")) -> ()  [unwired: 9 in, 2 out]
            n156 = local read "Output Filename (stem)"() -> (w226:path)
            n157 = Path To String(path=w226) -> (string=w227:string)
            n158 = Concatenate Strings(w227, "_summary.csv") -> (w229:string)
            n159 = String To Path(string=w229) -> (path=w225:path)
            n160 = Build Array (concatenate)(w208, w210) -> (w207:string[][])
            n161 = call-poly <vilib>:"Write Delimited Spreadsheet.vi"("file path (dialog if empty)"=w225, "2D data"=w207, "transpose? (no:F)"=FALSE, "delimiter (\\t)"="," ("delimiter (\\t)")) -> ()  [unwired: 10 in, 2 out]
          }
        }
      }
      event Timeout {
        # "If we are currently collecting \ndata, the user should not be \nable to change controls."
        n162 = event-data() -> ()  [unwired: 1 in, 3 out]
        n163 = local read "Running"() -> (w296:bool)
        n164 = case shown="False" w296 {
          tunnel: w295 -> [w301 _]
          tunnel: w294 -> [w300 _]
          tunnel: w293 -> [w299 _]
          tunnel: w292 -> [w298 _]
          frame False {
            w303 = T8."Disabled and Grayed Out" ("Disabled")
            w304 = T8."Enabled" ("Disabled")
            # "Allow user to adjust the position of the translation stage."
            # "In \"Reference\" mode, the program should store \ndata in the reference indicators. In the \"Sample\" \nmode, the sample indicators should be used. \nThis allows the calculation of the dichroic ratio, \nand hence the dipole orientation."
            n165 = local read "Save Measurements?"() -> (w305:bool)
            n166 = Equal?(x="Data Collection Mode", y=enum32{"Reference", "Sample"}."Sample") -> (x = y?=w308:bool)
            n167 = Select(t=w303, s=w308, f=w304) -> ()  [unwired: 1 out]
            n168 = Select(t=w304, s=w308, f=w303) -> ()  [unwired: 1 out]
            n169 = Select(t=w304, s=w305, f=w303) -> (s? t:f=w306:T8)
            n170 = property on="Output Filename (stem)" class="Path"("DisabledEnum"=w306) -> ()  [unwired: 2 in, 2 out]
            n171 = for {
              N: 100 -> [_]
              shift-right: [w315] -> _
              shift-left: MCTypedef."idle" -> [w316]
              tunnel: w301 -> [w313]
              tunnel: w300 -> [w312]
              tunnel: w299 -> [w311]
              tunnel: w298 -> [w310]
              n172 = case shown="\"idle\", Default" w316 {
                tunnel: [w317 MCTypedef."idle" MCTypedef."idle" MCTypedef."idle"] -> w315
                tunnel: [_ w367 w400 w436] -> w314
                tunnel: w312 -> [_ w366 w399 w435]
                tunnel: w313 -> [_ w365 w398 w434]
                tunnel: w310 -> [w324 _ _ _]
                tunnel: w311 -> [w322 _ _ _]
                tunnel: [w323 _ _ _] -> _
                frame "idle", Default {
                  n173 = flat-sequence {
                    tunnel: w324 -> [w340]
                    tunnel: w322 -> [w335]
                    tunnel: [w339] -> w321
                    tunnel: [MCTypedef."clear" ("t")] -> w320
                    tunnel: ["clear"] -> w319
                    tunnel: [w326] -> w318
                    tunnel: [w359] -> w323
                    tunnel: w321 -> [w359]
                    tunnel: w320 -> [w357]
                    tunnel: w319 -> [w358]
                    tunnel: w318 -> [w356]
                    tunnel: [w355] -> w317
                    frame #0 {
                      w332 = T15 [enum."DOWN"] items=["0", "1", "2", "3", "4", "5", "6", "7", "8", "9", "A", "B", "C", "D", "E", "F", "G", "H", "I", "J", "K", "L", "M", "N", "O", "P", "Q", "R", "S", "T", "U", "V", "W", "X", "Y", "Z", "F1", "F2", "F3", "F4", "F5", "F6", "F7", "F8", "F9", "F10", "F11", "F12", "F13", "F14", "F15", "ADD", "BACK", "BACKSLASH", "CAPITAL", "COMMA", "DECIMAL", "DELETE", "DIVIDE", "DOWN", "END", "EQUALS", "ESCAPE", "GRAVE (`)", "HOME", "INSERT", "LBRACKET", "LCONTROL", "LEFT", "L ALT", "LSHIFT", "LWIN", "MINUS", "MULTIPLY", "NEXT", "NUMLOCK", "NUMPAD_0", "NUMPAD_1", "NUMPAD_2", "NUMPAD_3", "NUMPAD_4", "NUMPAD_5", "NUMPAD_6", "NUMPAD_7", "NUMPAD_8", "NUMPAD_9", "PAUSE", "PERIOD", "PRIOR (PG UP)", "RBRACKET", "RCONTROL", "RETURN", "RIGHT", "R ALT", "RSHIFT", "RWIN", "SCROLL", "SEMICOLON", "SLASH", "SPACE", "SUBTRACT", "TAB", "UP", "ENTER (num pad)", "' (quote)"] ("y")
                      w338 = T15 [enum."UP"] items=["0", "1", "2", "3", "4", "5", "6", "7", "8", "9", "A", "B", "C", "D", "E", "F", "G", "H", "I", "J", "K", "L", "M", "N", "O", "P", "Q", "R", "S", "T", "U", "V", "W", "X", "Y", "Z", "F1", "F2", "F3", "F4", "F5", "F6", "F7", "F8", "F9", "F10", "F11", "F12", "F13", "F14", "F15", "ADD", "BACK", "BACKSLASH", "CAPITAL", "COMMA", "DECIMAL", "DELETE", "DIVIDE", "DOWN", "END", "EQUALS", "ESCAPE", "GRAVE (`)", "HOME", "INSERT", "LBRACKET", "LCONTROL", "LEFT", "L ALT", "LSHIFT", "LWIN", "MINUS", "MULTIPLY", "NEXT", "NUMLOCK", "NUMPAD_0", "NUMPAD_1", "NUMPAD_2", "NUMPAD_3", "NUMPAD_4", "NUMPAD_5", "NUMPAD_6", "NUMPAD_7", "NUMPAD_8", "NUMPAD_9", "PAUSE", "PERIOD", "PRIOR (PG UP)", "RBRACKET", "RCONTROL", "RETURN", "RIGHT", "R ALT", "RSHIFT", "RWIN", "SCROLL", "SEMICOLON", "SLASH", "SPACE", "SUBTRACT", "TAB", "UP", "ENTER (num pad)", "' (quote)"] ("y")
                      n174 = call-poly <vilib>:"Acquire Input Data.vi"("device ID"=w340, "error in (no error)"=w335) -> ("device ID"=w339:refnum<k1>, "keys pressed"=w331:T15)  [unwired: 15 in, 1 out]
                      n175 = Equal?(x=w331, y=w338) -> (x = y?=w337:bool[])
                      n176 = Index Array(array=w337, index=0) -> (element=w330:bool)
                      n177 = Equal?(x=w331, y=w332) -> (x = y?=w333:bool[])
                      n178 = Index Array(array=w333, index=0) -> (element=w329:bool)
                      n179 = Select(t=1, s=w330, f=0) -> (s? t:f=w349:i32)
                      n180 = Select(t=2, s=w329, f=0) -> (s? t:f=w348:i32)
                      n181 = Or(x=w349, y=w348) -> (x .or. y?=w347:i32)
                      n182 = Equal?(x=w347, y=1) -> (x = y?=w345:bool)
                      n183 = Select(t=MCTypedef."forward", s=w345, f=MCTypedef."reverse") -> (s? t:f=w341:T9)
                      n184 = Exclusive Or(1:w329, 2:w330) -> (0:w354:bool)
                      n185 = Select(t=w341, s=w354, f=MCTypedef."idle") -> (s? t:f=w326:T9)
                    }
                    frame #1 {
                      n186 = Select(t=w357, s=w358, f=w356) -> (s? t:f=w355:T9)
                    }
                  }
                  n187 = Wait (ms)(milliseconds to wait=u32 50) -> ()  [unwired: 1 out]
                }
                frame "forward" {
                  n188 = Multiply(x="sp33d", y=0.1) -> (x*y=w362:dbl)
                  n189 = Format Into String(format string="%1.2f", w362) -> (resulting string=w360:string)  [unwired: 2 in, 1 out]
                  n190 = flat-sequence {
                    tunnel: [w382] -> w372
                    tunnel: [w381] -> w371
                    tunnel: w366 -> [w375]
                    tunnel: w365 -> [w374]
                    tunnel: w360 -> [w373]
                    tunnel: w372 -> [w388]
                    tunnel: w371 -> [w387]
                    tunnel: [w386] -> w370
                    tunnel: [w385] -> w369
                    tunnel: w370 -> [w391]
                    tunnel: w369 -> [w392]
                    tunnel: [w390] -> _
                    tunnel: [w389] -> w367
                    frame #0 {
                      (unwired) "1.0" ("string")
                      n191 = call <vilib>:"Space Constant.vi"() -> ("String"=w376:string)
                      n192 = Concatenate Strings("jog2" ("string"), w376, w373, "\r", "\n") -> (w377:string)
                      n193 = VISA Write(VISA resource name=w375, write buffer=w377, error in (no error)=w374) -> (VISA resource name out=w382:refnum<visa-resource-name>, error out=w381:errorcluster)  [unwired: 1 out]
                    }
                    frame #1 {
                      n194 = VISA Read(VISA resource name=w388, byte count=u32 1024, error in (no error)=w387) -> (VISA resource name out=w386:refnum<visa-resource-name>, read buffer=→"read buffer":string, error out=w385:errorcluster)  [unwired: 1 out]
                    }
                    frame #2 {
                      n195 = VISA Flush I/O Buffer(VISA resource name=w391, error in (no error)=w392) -> (VISA resource name out=w390:refnum<visa-resource-name>, error out=w389:errorcluster)  [unwired: 1 in]
                    }
                  }
                }
                frame "reverse" {
                  n196 = local read "sp33d"() -> (w394:dbl)
                  n197 = Multiply(x=w394, y=-0.1) -> (x*y=w397:dbl)
                  n198 = Format Into String(format string="%1.2f", w397) -> (resulting string=w393:string)  [unwired: 2 in, 1 out]
                  n199 = flat-sequence {
                    tunnel: [w415] -> w405
                    tunnel: [w414] -> w404
                    tunnel: w399 -> [w408]
                    tunnel: w398 -> [w407]
                    tunnel: w393 -> [w406]
                    tunnel: w405 -> [w421]
                    tunnel: w404 -> [w420]
                    tunnel: [w419] -> w403
                    tunnel: [w418] -> w402
                    tunnel: w403 -> [w424]
                    tunnel: w402 -> [w425]
                    tunnel: [w423] -> _
                    tunnel: [w422] -> w400
                    frame #0 {
                      n200 = call <vilib>:"Space Constant.vi"() -> ("String"=w409:string)
                      n201 = Concatenate Strings("jog2" ("string"), w409, w406, "\r", "\n") -> (w410:string)
                      n202 = VISA Write(VISA resource name=w408, write buffer=w410, error in (no error)=w407) -> (VISA resource name out=w415:refnum<visa-resource-name>, error out=w414:errorcluster)  [unwired: 1 out]
                    }
                    frame #1 {
                      n203 = VISA Read(VISA resource name=w421, byte count=u32 1024, error in (no error)=w420) -> (VISA resource name out=w419:refnum<visa-resource-name>, read buffer=w416:string, error out=w418:errorcluster)  [unwired: 1 out]
                      n204 = local write "read buffer"(w416) -> ()
                    }
                    frame #2 {
                      n205 = VISA Flush I/O Buffer(VISA resource name=w424, error in (no error)=w425) -> (VISA resource name out=w423:refnum<visa-resource-name>, error out=w422:errorcluster)  [unwired: 1 in]
                    }
                  }
                }
                frame "clear" {
                  n206 = flat-sequence {
                    tunnel: [w446] -> w429
                    tunnel: [w445] -> w427
                    tunnel: w435 -> [w441]
                    tunnel: w434 -> [w440]
                    tunnel: w429 -> [w450]
                    tunnel: [w448] -> w428
                    tunnel: w427 -> [w449]
                    tunnel: [w447] -> w426
                    tunnel: w428 -> [w456]
                    tunnel: w426 -> [w455]
                    tunnel: [w454] -> w432
                    tunnel: [w451] -> w430
                    tunnel: [w465] -> w433
                    tunnel: w432 -> [w464]
                    tunnel: [w463] -> w431
                    tunnel: w430 -> [w457]
                    tunnel: w433 -> [w468]
                    tunnel: w431 -> [w469]
                    tunnel: [w467] -> _
                    tunnel: [w466] -> w436
                    frame #0 {
                      n207 = call <vilib>:"Space Constant.vi"() -> ("String"=w442:string)
                      n208 = Concatenate Strings("stop2" ("string"), w442, "\r", "\n") -> (w443:string)
                      n209 = VISA Write(VISA resource name=w441, write buffer=w443, error in (no error)=w440) -> (VISA resource name out=w446:refnum<visa-resource-name>, error out=w445:errorcluster)  [unwired: 1 out]
                    }
                    frame #1 {
                      n210 = VISA Flush I/O Buffer(VISA resource name=w450, error in (no error)=w449) -> (VISA resource name out=w448:refnum<visa-resource-name>, error out=w447:errorcluster)  [unwired: 1 in]
                    }
                    frame #2 {
                      n211 = VISA Read(VISA resource name=w456, byte count=u32 1024, error in (no error)=w455) -> (VISA resource name out=w451:refnum<visa-resource-name>, read buffer=w452:string, error out=w454:errorcluster)  [unwired: 1 out]
                      n212 = local write "read buffer"(w452) -> ()
                    }
                    frame #3 {
                      n213 = call <vilib>:"Space Constant.vi"() -> ("String"=w460:string)
                      n214 = Concatenate Strings("*cls" ("string"), w460, "\r", "\n") -> (w458:string)
                      n215 = VISA Write(VISA resource name=w457, write buffer=w458, error in (no error)=w464) -> (VISA resource name out=w465:refnum<visa-resource-name>, error out=w463:errorcluster)  [unwired: 1 out]
                    }
                    frame #4 {
                      n216 = VISA Flush I/O Buffer(VISA resource name=w468, error in (no error)=w469) -> (VISA resource name out=w467:refnum<visa-resource-name>, error out=w466:errorcluster)  [unwired: 1 in]
                    }
                  }
                }
              }
              "error out" <- w314
            }
          }
          frame True {
          }
        }
      }
      event "Measure Dark Current": Value Change {
        n217 = event-data() -> ("NewVal"=w472:bool)  [unwired: 1 in, 5 out]
        n218 = case shown="True" w472 {
          tunnel: w471 -> [_ w478]
          tunnel: w470 -> [_ w477]
          frame False {
          }
          frame True {
            n219 = flat-sequence {
              tunnel: w478 -> [w486]
              tunnel: w477 -> [w485]
              tunnel: [w482] -> w476
              tunnel: [w481] -> w475
              tunnel: w476 -> [_]
              tunnel: w475 -> [_]
              tunnel: [w491] -> w474
              tunnel: [w489] -> w473
              tunnel: w474 -> [w512]
              tunnel: w473 -> [w511]
              frame #0 {
                w479 = T8."Disabled and Grayed Out" ("Disabled")
                # "Close the shutter."
                n220 = call "LJUD_eDAC.vi"("Handle In"=w486, "Channel"=0, "Voltage"=0.0, "error in"=w485) -> ("Handle Out"=w482:i32, "error out"=w481:errorcluster)  [unwired: 10 in]
                n221 = Wait (ms)(milliseconds to wait=u32 2000) -> ()  [unwired: 1 out]
                n222 = property on="Measure Dark Current" class="Bool"("DisabledEnum"=w479) -> ()  [unwired: 2 in, 2 out]
                n223 = property on="Data Collection Mode" class="RadioBtnsControl (strict)"("DisabledEnum"=w479) -> ()  [unwired: 2 in, 2 out]
                n224 = property on="Collect Data" class="Bool (strict)"("DisabledEnum"=w479) -> ()  [unwired: 2 in, 2 out]
                n225 = property on="Save Measurements?" class="Bool (strict)"("DisabledEnum"=w479) -> ()  [unwired: 2 in, 2 out]
                n226 = property on="Output Filename (stem)" class="Path"("DisabledEnum"=w479) -> ()  [unwired: 2 in, 2 out]
                n227 = property on="Experimental Parameters" class="Clust (strict)"("DisabledEnum"=w479) -> ()  [unwired: 2 in, 2 out]
                n228 = property on="Export Data" class="Bool"("DisabledEnum"=w479) -> ()  [unwired: 2 in, 2 out]
              }
              frame #1 {
                w487 = "..\\MeasureDarkCurrent.vi" ("name or relative path")
                # "Signal dark current."
                # "Reference dark current."
                # "Measure dark current."
                n229 = Current VI's Path() -> (path=w488:path)
                n230 = Build Path(base path=w488, name or relative path=w487) -> (appended path=w500:path)
                n231 = Build Path(base path=w488, name or relative path=w487) -> (appended path=w510:path)
                n232 = Compound Arithmetic op=OR(64 ("options"), 256 ("options")) -> (w497:i32)
                n233 = Compound Arithmetic op=OR(64 ("options"), 256 ("options")) -> (w495:i32)
                n234 = Open VI Reference(type specifier VI Refnum (for type only)=refnum<vi> refnum, vi path=w500, options=w495) -> (vi reference=w502:refnum<vi>, error out=w503:errorcluster)  [unwired: 3 in]
                n235 = Open VI Reference(type specifier VI Refnum (for type only)=refnum<vi> refnum, vi path=w510, options=w497) -> (vi reference=w506:refnum<vi>, error out=w505:errorcluster)  [unwired: 3 in]
                n236 = call-by-ref "Start Asynchronous Call"(reference=w502, error in=w503, "Multimeter GPIB Address"="23", "Amplifier"=refnum<visa-resource-name> "COM4") -> ()  [unwired: 7 in, 4 out]
                n237 = call-by-ref "Start Asynchronous Call"(reference=w506, error in=w505, "Multimeter GPIB Address"="22", "Amplifier"=refnum<visa-resource-name> "COM3") -> ()  [unwired: 7 in, 4 out]
                n238 = call-by-ref "Wait On Asynchronous Call"(reference=w502, error in=w503) -> (reference out=w489:refnum<vi>, "Amplifier Settings"=→"Signal Amplifier Settings":T3)  [unwired: 9 in, 2 out]
                n239 = call-by-ref "Wait On Asynchronous Call"(reference=w506, error in=w505) -> (reference out=w491:refnum<vi>, "Amplifier Settings"=→"Reference Amplifier Settings":T3)  [unwired: 9 in, 2 out]
              }
              frame #2 {
                w513 = T8."Enabled" ("Disabled")
                # "Enable UI elements."
                n240 = Close Reference(reference=w512) -> ()  [unwired: 1 in, 1 out]
                n241 = Close Reference(reference=w511) -> ()  [unwired: 1 in, 1 out]
                n242 = invoke on="Measure Dark Current" class="Bool" method="Reinit To Default"() -> ()  [unwired: 3 in, 3 out]
                n243 = property on="Measure Dark Current" class="Bool"("DisabledEnum"=w513) -> ()  [unwired: 2 in, 2 out]
                n244 = property on="Data Collection Mode" class="RadioBtnsControl (strict)"("DisabledEnum"=w513) -> ()  [unwired: 2 in, 2 out]
                n245 = property on="Collect Data" class="Bool (strict)"("DisabledEnum"=w513) -> ()  [unwired: 2 in, 2 out]
                n246 = property on="Save Measurements?" class="Bool (strict)"("DisabledEnum"=w513) -> ()  [unwired: 2 in, 2 out]
                n247 = property on="Output Filename (stem)" class="Path"("DisabledEnum"=w513) -> ()  [unwired: 2 in, 2 out]
                n248 = property on="Experimental Parameters" class="Clust (strict)"("DisabledEnum"=w513) -> ()  [unwired: 2 in, 2 out]
                n249 = property on="Export Data" class="Bool"("DisabledEnum"=w513) -> ()  [unwired: 2 in, 2 out]
              }
            }
          }
        }
      }
    }
  }
